vi "Suggest new Window Name.vi"(11 "windows in":T1[](array[typedef])) -> (3 "suggested name":string)   [LabVIEW 2013, in "Engine Simulation Toolkit System Explorer.lvlib"]
uses:
  Engine Simulation Toolkit System Explorer.lvlib
  Event Timing Window.ctl
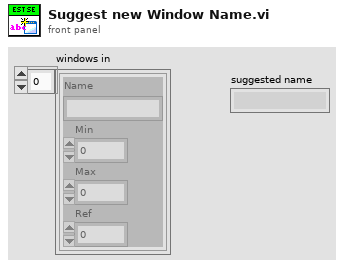
[diagram p1: front panel]
types:
  T1 = typedef "Engine Simulation Toolkit System Explorer.lvlib/Event Timing Window.ctl" = cluster{"Name":string, "Min":dbl, "Max":dbl, "Ref":dbl}
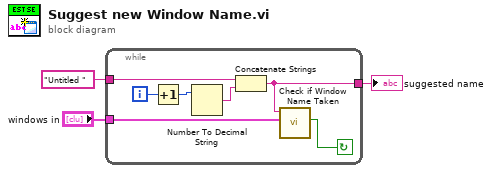
[diagram p0: block diagram]
diagram:
  n1 = while {
    tunnel: "windows in" -> [w10]
    tunnel: "Untitled " ("name") -> [w9]
    tunnel: [w5] -> w1
    i -> [w8]
    stop <- w4 continue-if-true
    n2 = Increment(x=w8) -> (x+1=w7:i32)
    n3 = Number To Decimal String(number=w7) -> (decimal integer string=w6:string)  [unwired: 1 in]
    n4 = Concatenate Strings(w9, w6) -> (w5:string)
    n5 = call "Check if Window Name Taken.vi"("windows in"=w10, "name"=w5) -> ("taken"=w4:bool)  [unwired: 9 in]
  }
  "suggested name" <- w1
